vi "HFRI software v11.vi"() -> ()   [LabVIEW 2019]
doc: "I. Description:\nThis example demonstrates how to output a finite number of voltage samples to an Analog Output Channel using an internal sample clock.\n\nII. Instructions for Running:\n1. Select the Physical Channel to correspond to where your signal is output on the DAQ device.\n2. Enter the Minimum and Maximum Voltage Ranges\n3. Specify the Desired Frequency of the output Waveform\n4. Enter the Waveform Information. See the documentation of the Waveform Buffer Generation SubVI for information on each parameter.\n\nIII. Block Diagram Steps:\n1. Create an Analog Output Voltage Channel.\n2. Call the DAQmx Timing (Use Waveform) VI which sets the sample clock rate based on the input waveform parameters, and set the sample mode to finite.\n3. Use the Write VI to Generate Multiple Samples to 1 Channel on the Data Acquisition Card. The auto start parameter is set to False, so the Start VI must explicitly be called to begin the Voltage Generation. \n4. Call the Start VI.\n5. Call the Wait Until Done VI, with a time limit of 10s.\n6. Call the Clear Task VI to clear the Task.\n7. Use the popup dialog box to display an error or warning if any.\n\nIV. I/O Connections Overview:\nMake sure your signal output terminal matches the Physical Channel I/O Control. For further connection information, refer to your hardware reference manual."
uses:
  C:/Temp/LabVIEW code/My droplet dispenser v11/Thorlabs.MotionControl.Controls.dll
  Thorlabs.MotionControl.Controls.dll
  C:/Temp/LabVIEW code/My droplet dispenser v11/ThorLabs.MotionControl.KCube.DCServoCLI.dll
  ThorLabs.MotionControl.KCube.DCServoCLI.dll
  <vilib>/DAQmx/write.llb/DAQmx Write (Analog 1D DBL 1Chan NSamp).vi
  5523896e-86ad-4b15-8550-5345652715c0.vi
  bf729f80-54d8-4e4c-bc1d-2b91bc905261.vi
  62c6f4b6-6490-4211-b8e5-8e663925be07.vi
  aa49ca9c-dec6-4f7c-ae92-68b6a477d75c.vi
  0b159907-7b32-4793-b7df-302a2670322c.vi
  bf0824da-a9b2-4ed7-8de6-d95a412e2ac0.vi
  <vilib>/DAQmx/miscellaneous.llb/DAQmx Fill In Error Info.vi
  <vilib>/DAQmx/create/channels.llb/DAQmx Create Channel (CO-Pulse Generation-Frequency).vi
  <vilib>/DAQmx/configure/timing.llb/DAQmx Timing (Implicit).vi
  <vilib>/DAQmx/create/channels.llb/DAQmx Create Channel (AO-Voltage-Basic).vi
  <vilib>/DAQmx/configure/timing.llb/DAQmx Timing (Sample Clock).vi
panel:
  in  "waitTimeout":i32=1000
  in  "KCubeDCServoControl":refnum<k24>(container)
  in  "Acceleration  / mm/s2":dbl=4.0 min=0.0 max=4.0
  in  "Velocity / mm/s":dbl=2.6 min=0.0 max=2.6
  in  "Step size / mm":dbl
  in  "Direction":i32(ring)=1 items=["Forward"=1, "Backward"=2]
  in  "?":bool
  in  "Capture":bool
  in  "Flash\ndummy":bool
  in  "Frequency (Hz)":dbl=10.0 min=0.0 step=0.1
  in  "Dispense":bool
  in  "Width / us":dbl=35.0
  in  "Amplitude / V":dbl=5.0
  in  "Amplitude / V":dbl
  in  "Width / us":dbl
  out "Pulse waveform":dbl[](array[numeric])
  out "Waveform Graph":dbl[](graph)
  # "High Frame Rate Imaging System"
  # "Actual pulse"
  # "Dispensing controls"
  # "Dummy pulse"
  # "Translation stage controls"
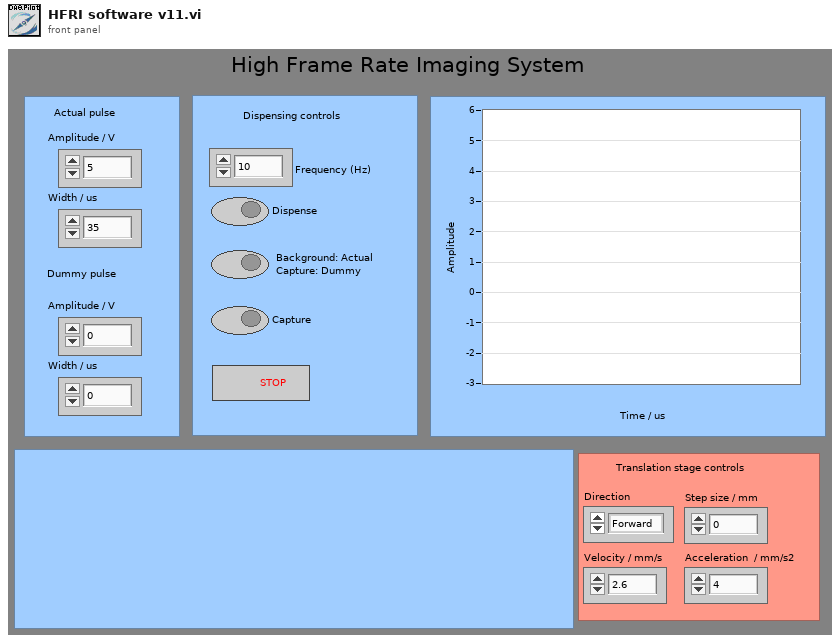
[diagram p1: front panel]
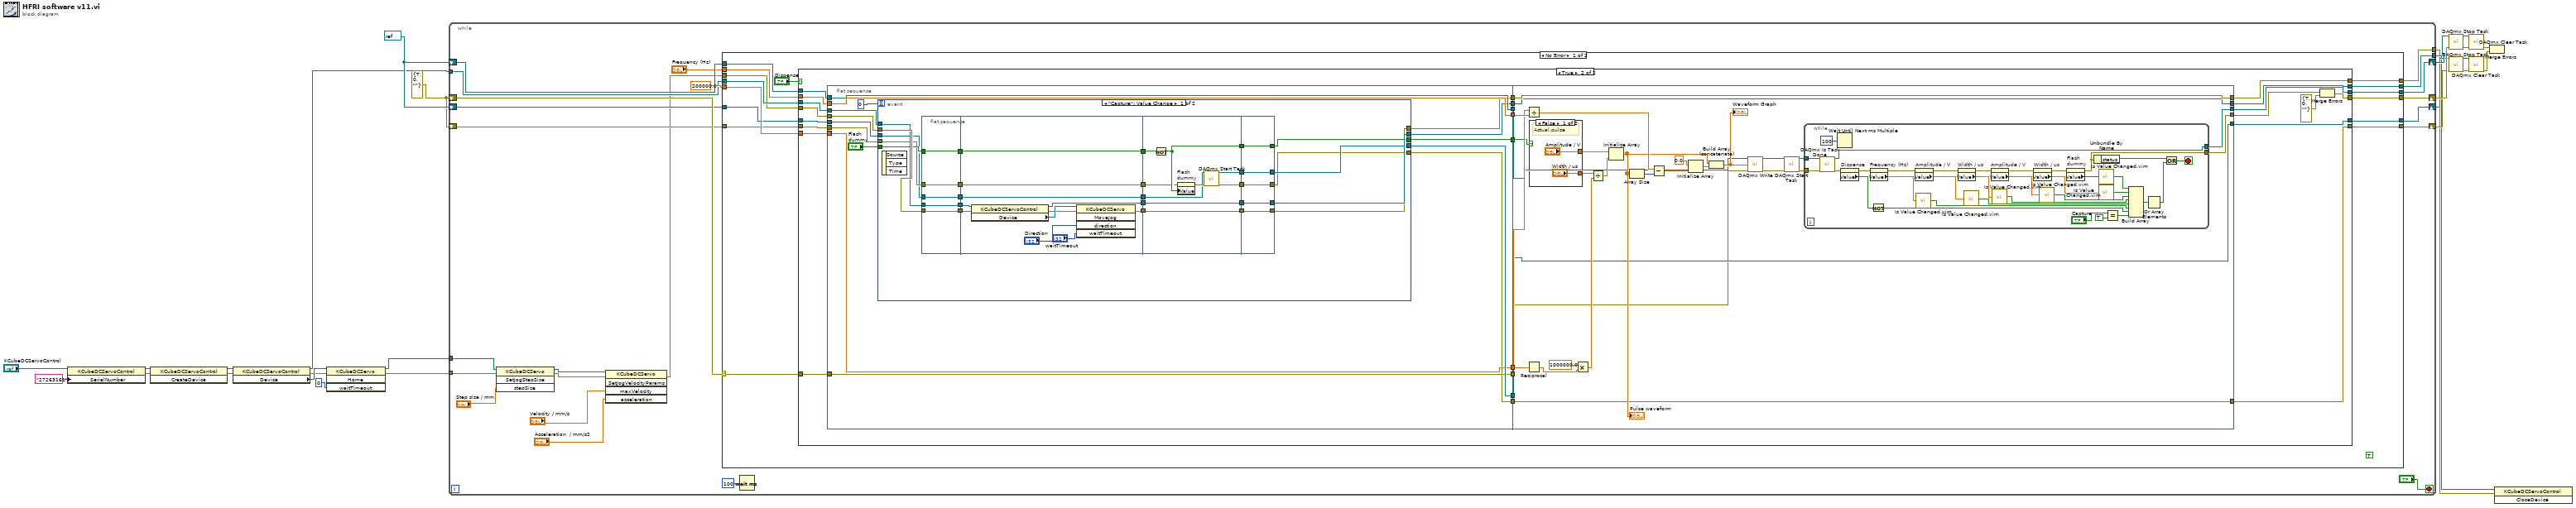
[diagram p0: block diagram]
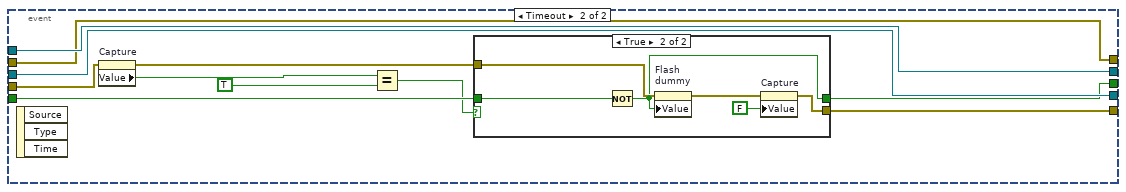
[diagram p3: hidden frame]
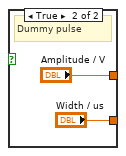
[diagram p5: hidden frame]
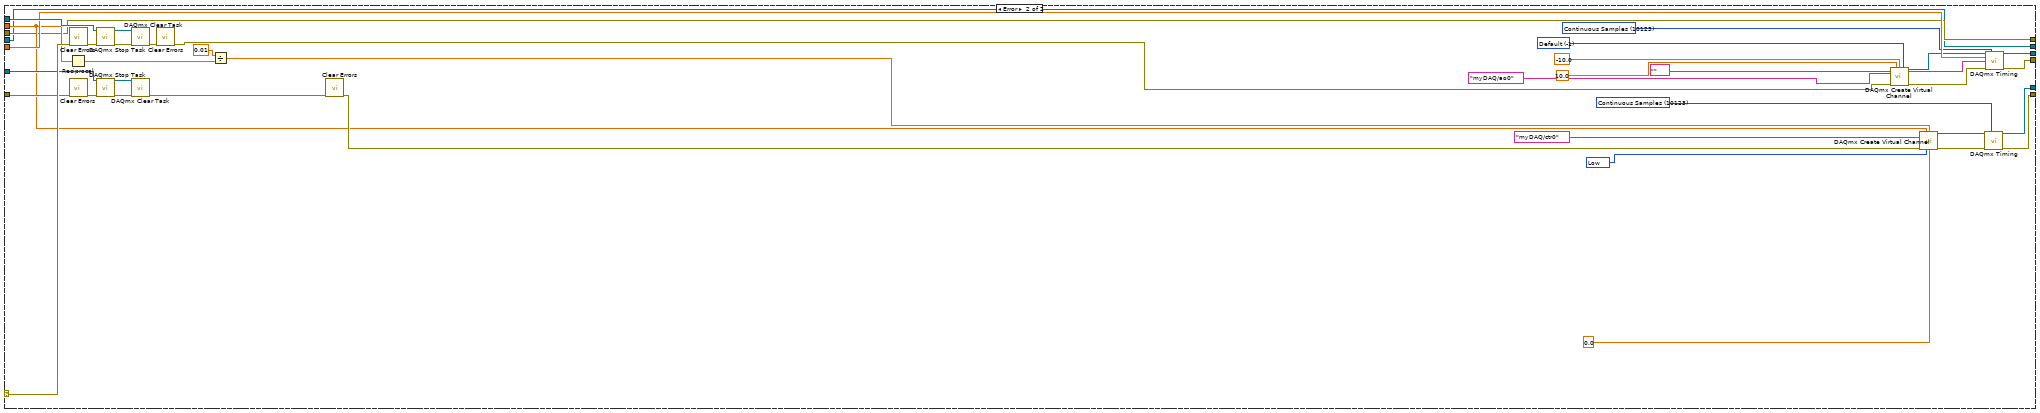
[diagram p6: hidden frame]
diagram:
  w16 = refnum<k21> refnum ("task/channels in")
  w15 = errorcluster {"status"=TRUE, "code"=0, "source"=""} ("error in")
  n1 = property class="KCubeDCServoControl"(reference="KCubeDCServoControl", "SerialNumber"="27263161") -> (reference out=w11:refnum<k24>, error out=w12:errorcluster)  [unwired: 1 in]
  n2 = invoke class="KCubeDCServoControl" method="CreateDevice"(reference=w11, error in=w12) -> (reference out=w13:refnum<k24>, error out=w14:errorcluster)  [unwired: 1 in, 1 out]
  n3 = property class="KCubeDCServoControl"(reference=w13, error in=w14) -> (reference out=w9:refnum<k24>, error out=w2:errorcluster, "Device"=w3:refnum<k24>)
  n4 = invoke class="KCubeDCServo" method="Home"(reference=w3, error in=w2, "waitTimeout"=0) -> (reference out=w1:refnum<k24>, error out=w4:errorcluster)  [unwired: 1 in, 2 out]
  n5 = while {
    shift-right: [w47] -> w26
    shift-left: w16 -> [w48]
    shift-right: [w46] -> w25
    shift-left: w15 -> [w44]
    shift-right: [w42] -> w19
    shift-left: w16 -> [w40]
    shift-right: [w41] -> w21
    shift-left: w15 -> [w39]
    tunnel: w9 -> [w37]
    tunnel: w4 -> [w33]
    tunnel: [w36] -> w6
    tunnel: [w35] -> w5
    tunnel: w1 -> [w34]
    stop <- "?" stop-if-true
    n6 = invoke class="KCubeDCServo" method="SetJogStepSize"(reference=w34, error in=w33, "stepSize"="Step size / mm") -> (reference out=w31:refnum<k24>, error out=w32:errorcluster)  [unwired: 1 in, 2 out]
    n7 = invoke class="KCubeDCServo" method="SetJogVelocityParams"(reference=w31, error in=w32, "maxVelocity"="Velocity / mm/s", "acceleration"="Acceleration  / mm/s2") -> (error out=w30:errorcluster)  [unwired: 1 in, 4 out]
    n8 = case shown="No Error" w44 {
      selector: w44 -> [w64 w285]
      tunnel: [w62 w288] -> w47
      tunnel: [w61 w287] -> w46
      tunnel: w48 -> [w63 w286]
      tunnel: 200000.0 ("rate") -> [w60 w284]
      tunnel: [w58 w253] -> w42
      tunnel: [w57 w254] -> w41
      tunnel: w40 -> [w56 w265]
      tunnel: w39 -> [w55 w266]
      tunnel: "Frequency (Hz)" -> [w54 w252]
      tunnel: w37 -> [w53 w250]
      tunnel: w30 -> [w52 w251]
      tunnel: [w51 w250] -> w36
      tunnel: [w50 w251] -> w35
      frame No Error {
        (unwired) TRUE
        n9 = case shown="True" "Dispense" {
          tunnel: w63 -> [w69 w79]
          tunnel: w64 -> [w70 w81]
          tunnel: [w69 w93] -> w62
          tunnel: [w70 w94] -> w61
          tunnel: w60 -> [_ w85]
          tunnel: [w67 w82] -> w57
          tunnel: [w68 w83] -> w58
          tunnel: w56 -> [w68 w91]
          tunnel: w55 -> [w67 w90]
          tunnel: w54 -> [_ w87]
          tunnel: w53 -> [w65 w76]
          tunnel: w52 -> [w66 w75]
          tunnel: [w65 w72] -> w51
          tunnel: [w66 w71] -> w50
          frame False {
          }
          frame True {
            n10 = flat-sequence {
              tunnel: w91 -> [w105]
              tunnel: w90 -> [w104]
              tunnel: [w110] -> w89
              tunnel: [w109] -> w88
              tunnel: w87 -> [w107]
              tunnel: [w107] -> w86
              tunnel: w85 -> [w106]
              tunnel: [w106] -> w84
              tunnel: w81 -> [w103]
              tunnel: [w103] -> w80
              tunnel: w79 -> [w102]
              tunnel: [w102] -> w78
              tunnel: [w100] -> w77
              tunnel: w76 -> [w99]
              tunnel: w75 -> [w98]
              tunnel: [w97] -> w74
              tunnel: [w96] -> w73
              tunnel: [w210] -> w93
              tunnel: [w209] -> w92
              tunnel: w89 -> [w193]
              tunnel: w88 -> [w192]
              tunnel: w86 -> [w195]
              tunnel: w84 -> [w194]
              tunnel: [w193] -> w83
              tunnel: [w192] -> w82
              tunnel: w80 -> [w191]
              tunnel: w78 -> [w190]
              tunnel: w77 -> [w187]
              tunnel: w74 -> [w185]
              tunnel: w73 -> [w186]
              tunnel: [w186] -> w71
              tunnel: [w185] -> w72
              frame #0 {
                n11 = event shown="[0] \"Capture\": Value Change" {
                  selector: _ -> [_ _]
                  dyn-events: _ -> [_ _]
                  timeout: 0 -> [_ _]
                  tunnel: w105 -> [w122 w176]
                  tunnel: w104 -> [w123 w175]
                  tunnel: [w125 w171] -> w109
                  tunnel: [w126 w176] -> w110
                  tunnel: "Flash\ndummy" -> [w127 w170]
                  tunnel: [w129 w169] -> w100
                  tunnel: w99 -> [w132 w167]
                  tunnel: w98 -> [w133 w166]
                  tunnel: [w135 w167] -> w97
                  tunnel: [w134 w166] -> w96
                  event "Capture": Value Change {
                    n12 = event-data() -> ()  [unwired: 1 in, 3 out]
                    n13 = flat-sequence {
                      tunnel: w122 -> [w136]
                      tunnel: w123 -> [w137]
                      tunnel: w127 -> [w138]
                      tunnel: w132 -> [w139]
                      tunnel: w133 -> [w140]
                      tunnel: [w140] -> w115
                      tunnel: [w139] -> w114
                      tunnel: [w138] -> w113
                      tunnel: [w137] -> w112
                      tunnel: [w136] -> w111
                      tunnel: [w149] -> w131
                      tunnel: [w148] -> w130
                      tunnel: [w143] -> w128
                      tunnel: [w142] -> w124
                      tunnel: [w141] -> w121
                      tunnel: w115 -> [w147]
                      tunnel: w114 -> [w146]
                      tunnel: w113 -> [w143]
                      tunnel: w112 -> [w142]
                      tunnel: w111 -> [w141]
                      tunnel: w131 -> [w160]
                      tunnel: w130 -> [w159]
                      tunnel: w128 -> [w157]
                      tunnel: w124 -> [w153]
                      tunnel: w121 -> [w152]
                      tunnel: [w160] -> w120
                      tunnel: [w159] -> w119
                      tunnel: [w158] -> w118
                      tunnel: [w155] -> w117
                      tunnel: [w154] -> w116
                      tunnel: [w161] -> w125
                      tunnel: [w162] -> w126
                      tunnel: [w163] -> w129
                      tunnel: [w164] -> w134
                      tunnel: [w165] -> w135
                      tunnel: w120 -> [w165]
                      tunnel: w119 -> [w164]
                      tunnel: w118 -> [w163]
                      tunnel: w117 -> [w162]
                      tunnel: w116 -> [w161]
                      frame #0 {
                      }
                      frame #1 {
                        n14 = property class="KCubeDCServoControl"(reference=w146, error in=w147) -> (reference out=w149:refnum<k24>, error out=w150:errorcluster, "Device"=w151:refnum<k24>)
                        n15 = invoke class="KCubeDCServo" method="MoveJog"(reference=w151, error in=w150, "direction"="Direction", "waitTimeout"="waitTimeout") -> (error out=w148:errorcluster)  [unwired: 1 in, 4 out]
                      }
                      frame #2 {
                        n16 = Not(x=w157) -> (.not. x?=w158:bool)
                        n17 = property on="Flash\ndummy" class="Bool (strict)"(error in=w153, "Value"=w158) -> (error out=w156:errorcluster)  [unwired: 1 in, 1 out]
                        n18 = call <vilib>:"DAQmx Start Task.vi"("task/channels in"=w152, "error in"=w156) -> ("task out"=w155:refnum<k21>, "error out"=w154:errorcluster)  [unwired: 12 in]
                      }
                      frame #3 {
                      }
                    }
                  }
                  event Timeout {
                    n19 = event-data() -> ()  [unwired: 1 in, 3 out]
                    n20 = property on="Capture" class="Bool (strict)"(error in=w175) -> (error out=w172:errorcluster, "Value"=w174:bool)  [unwired: 1 in, 1 out]
                    n21 = Equal?(x=w174, y=TRUE) -> (x = y?=w168:bool)
                    n22 = case shown="True" w168 {
                      tunnel: w172 -> [w178 w184]
                      tunnel: [w178 w180] -> w171
                      tunnel: w170 -> [w177 w183]
                      tunnel: [w177 w182] -> w169
                      frame False {
                      }
                      frame True {
                        n23 = Not(x=w183) -> (.not. x?=w182:bool)
                        n24 = property on="Flash\ndummy" class="Bool (strict)"(error in=w184, "Value"=w182) -> (error out=w181:errorcluster)  [unwired: 1 in, 1 out]
                        n25 = property on="Capture" class="Bool (strict)"(error in=w181, "Value"=FALSE ("Capture")) -> (error out=w180:errorcluster)  [unwired: 1 in, 1 out]
                      }
                    }
                  }
                }
              }
              frame #1 {
                n26 = Divide(x=w194, y=w195) -> (x/y=w205:dbl)
                n27 = Reciprocal(x=w194) -> (1/x=w202:dbl)
                n28 = case shown="False" w187 {
                  tunnel: ["Amplitude / V" "Amplitude / V"] -> w207
                  tunnel: ["Width / us" "Width / us"] -> w208
                  frame False {
                    # "Actual pulse"
                  }
                  frame True {
                    # "Dummy pulse"
                  }
                }
                n29 = Multiply(x=1000000.0 ("y"), y=w202) -> (x*y=w203:dbl)
                n30 = Divide(x=w208, y=w203) -> (x/y=w198:dbl)
                n31 = Initialize Array(w207, w198) -> (w204:dbl[])
                "Pulse waveform" <- w204
                n32 = Array Size(array=w204) -> (size(s)=w201:i32)
                n33 = Subtract(x=w205, y=w201) -> (x-y=w199:dbl)
                n34 = Initialize Array(0.0 ("element"), w199) -> (w200:dbl[])
                n35 = Build Array (concatenate)(w204, w200) -> (w206:dbl[])
                "Waveform Graph" <- w206
                n36 = call-poly <vilib>:"DAQmx Write.vi"("task/channels in"=w190, "data"=w206, "error in"=w191) -> ("task out"=w189:refnum<k21>, "error out"=w188:errorcluster)  [unwired: 10 in, 1 out]
                n37 = call <vilib>:"DAQmx Start Task.vi"("task/channels in"=w189, "error in"=w188) -> ("task out"=w212:refnum<k21>, "error out"=w211:errorcluster)  [unwired: 12 in]
                n38 = while {
                  tunnel: w212 -> [w249]
                  tunnel: [w248] -> w210
                  tunnel: w211 -> [w247]
                  tunnel: [w232] -> w209
                  stop <- w245 stop-if-true
                  n39 = call <vilib>:"DAQmx Is Task Done.vi"("task/channels in"=w249, "error in"=w247) -> ("task out"=w248:refnum<k21>, "error out"=w220:errorcluster)  [unwired: 11 in, 1 out]
                  n40 = Wait Until Next ms Multiple(millisecond multiple=u32 100) -> ()  [unwired: 1 out]
                  n41 = property on="Dispense" class="Bool (strict)"(error in=w220) -> (error out=w230:errorcluster, "Value"=w235:bool)  [unwired: 1 in, 1 out]
                  n42 = property on="Frequency (Hz)" class="DigNum (strict)"(error in=w230) -> (error out=w242:errorcluster, "Value"=w244:dbl)  [unwired: 1 in, 1 out]
                  n43 = Not(x=w235) -> (.not. x?=w223:bool)
                  n44 = property on="Amplitude / V" class="DigNum (strict)"(error in=w242) -> (error out=w241:errorcluster, "Value"=w243:dbl)  [unwired: 1 in, 1 out]
                  n45 = call "Is Value Changed.vim"("value"=w244) -> ("changed or first call?"=w224:bool)
                  n46 = property on="Width / us" class="DigNum (strict)"(error in=w241) -> (error out=w239:errorcluster, "Value"=w240:dbl)  [unwired: 1 in, 1 out]
                  n47 = call "Is Value Changed.vim"("value"=w243) -> ("changed or first call?"=w225:bool)
                  n48 = property on="Amplitude / V" class="DigNum (strict)"(error in=w239) -> (error out=w238:errorcluster, "Value"=w237:dbl)  [unwired: 1 in, 1 out]
                  n49 = call "Is Value Changed.vim"("value"=w240) -> ("changed or first call?"=w226:bool)
                  n50 = property on="Width / us" class="DigNum (strict)"(error in=w238) -> (error out=w233:errorcluster, "Value"=w236:dbl)  [unwired: 1 in, 1 out]
                  n51 = call "Is Value Changed.vim"("value"=w237) -> ("changed or first call?"=w227:bool)
                  n52 = property on="Flash\ndummy" class="Bool (strict)"(error in=w233) -> (error out=w232:errorcluster, "Value"=w231:bool)  [unwired: 1 in, 1 out]
                  n53 = Unbundle By Name(w232) -> ("status"=w234:bool)
                  n54 = call "Is Value Changed.vim"("value"=w231) -> ("changed or first call?"=w229:bool)
                  n55 = call "Is Value Changed.vim"("value"=w236) -> ("changed or first call?"=w228:bool)
                  n56 = Equal?(x="Capture", y=TRUE) -> (x = y?=w217:bool)
                  n57 = Build Array(w229, w228, w227, w226, w225, w224, w223, w217) -> (w222:bool[])
                  n58 = Or Array Elements(Boolean array=w222) -> (logical OR=w221:bool)
                  n59 = Or(x=w234, y=w221) -> (x .or. y?=w245:bool)
                }
              }
            }
            n60 = Merge Errors(w92, errorcluster {"status"=TRUE, "code"=0, "source"=""} ("error in")) -> (w94:errorcluster)
          }
        }
      }
      frame Error {
        w257 = 10214 items=["High"=10192, "Low"=10214] ("idle state")
        w259 = 10123 items=["Finite Samples"=10178, "Continuous Samples"=10123, "Hardware Timed Single Point"=12522] ("sample mode")
        w277 = 10123 items=["Finite Samples"=10178, "Continuous Samples"=10123, "Hardware Timed Single Point"=12522] ("sample mode")
        w280 = -1 items=["Default"=-1, "RSE"=10083, "Differential"=10106, "Pseudodifferential"=12529] ("output terminal configuration")
        n61 = call <vilib>:"Clear Errors.vi"("error in (no error)"=w285) -> ("error out"=w273:errorcluster)  [unwired: 5 in, 1 out]
        n62 = Reciprocal(x=w252) -> (1/x=w261:dbl)
        n63 = call <vilib>:"Clear Errors.vi"("error in (no error)"=w266) -> ("error out"=w270:errorcluster)  [unwired: 5 in, 1 out]
        n64 = call <vilib>:"DAQmx Stop Task.vi"("task/channels in"=w286, "error in"=w273) -> ("task out"=w276:refnum<k21>, "error out"=w275:errorcluster)  [unwired: 12 in]
        n65 = call <vilib>:"DAQmx Stop Task.vi"("task/channels in"=w265, "error in"=w270) -> ("task out"=w267:refnum<k21>, "error out"=w268:errorcluster)  [unwired: 12 in]
        n66 = call <vilib>:"DAQmx Clear Task.vi"("task in"=w276, "error in"=w275) -> ("error out"=w274:errorcluster)  [unwired: 13 in]
        n67 = call <vilib>:"DAQmx Clear Task.vi"("task in"=w267, "error in"=w268) -> ("error out"=w269:errorcluster)  [unwired: 13 in]
        n68 = call <vilib>:"Clear Errors.vi"("error in (no error)"=w274) -> ("error out"=w272:errorcluster)  [unwired: 5 in, 1 out]
        n69 = Divide(x=0.01 ("low time"), y=w261) -> (x/y=w262:dbl)
        n70 = call <vilib>:"Clear Errors.vi"("error in (no error)"=w269) -> ("error out"=w255:errorcluster)  [unwired: 5 in, 1 out]
        n71 = call-poly <vilib>:"DAQmx Create Virtual Channel.vi"("maximum value"=10.0, "minimum value"=-10.0, "output terminal configuration"=w280, "physical channels"=tag "myDAQ/ao0", "error in"=w272) -> ("task out"=w279:refnum<k21>, "error out"=w278:errorcluster)  [unwired: 9 in]
        n72 = call-poly <vilib>:"DAQmx Create Virtual Channel.vi"("frequency"=w252, "duty cycle"=w262, "counter"=tag "myDAQ/ctr0", "error in"=w255, "idle state"=w257, "initial delay"=0.0) -> ("task out"=w263:refnum<k21>, "error out"=w264:errorcluster)  [unwired: 8 in]
        n73 = call-poly <vilib>:"DAQmx Timing.vi"("task/channels in"=w263, "sample mode"=w259, "error in"=w264) -> ("task out"=w253:refnum<k21>, "error out"=w254:errorcluster)  [unwired: 11 in]
        n74 = call-poly <vilib>:"DAQmx Timing.vi"("task/channels in"=w279, "sample mode"=w277, "rate"=w284, "source"=tag "", "error in"=w278) -> ("task out"=w288:refnum<k21>, "error out"=w287:errorcluster)  [unwired: 9 in]
      }
    }
    n75 = Wait (ms)(milliseconds to wait=u32 100) -> ()  [unwired: 1 out]
  }
  n76 = call <vilib>:"DAQmx Stop Task.vi"("task/channels in"=w26, "error in"=w25) -> ("task out"=w24:refnum<k21>, "error out"=w23:errorcluster)  [unwired: 12 in]
  n77 = call <vilib>:"DAQmx Stop Task.vi"("task/channels in"=w19, "error in"=w21) -> ("task out"=w22:refnum<k21>, "error out"=w20:errorcluster)  [unwired: 12 in]
  n78 = call <vilib>:"DAQmx Clear Task.vi"("task in"=w24, "error in"=w23) -> ("error out"=w18:errorcluster)  [unwired: 13 in]
  n79 = call <vilib>:"DAQmx Clear Task.vi"("task in"=w22, "error in"=w20) -> ("error out"=w17:errorcluster)  [unwired: 13 in]
  n80 = Merge Errors(w18, w17) -> ()  [unwired: 1 out]
  n81 = invoke class="KCubeDCServoControl" method="CloseDevice"(reference=w6, error in=w5) -> ()  [unwired: 1 in, 3 out]
